vi "Connect References to Bundle By Name.vi"(7 "Sources":refnum<vi>[](array[refnum]), 8 "error in":errorcluster, 9 "BBN Node":refnum<vi>, 10 "SubVI Output Terminal":refnum<vi>) -> (0 "error out":errorcluster, 2 "New Wires":refnum<vi>[](array[refnum]))   [LabVIEW 2015, in "Build Cluster of References__RCF.lvlib"]
doc: "Connects several references to the inputs of a Bundle By Name primitive and aligns them."
uses:
  Build Cluster of References__RCF.lvlib
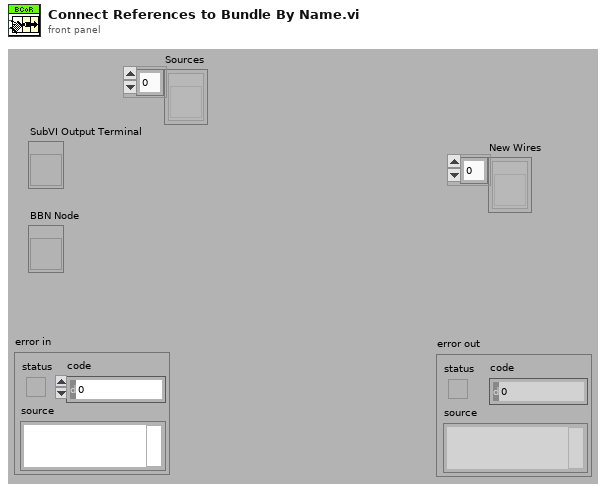
[diagram p1: front panel]
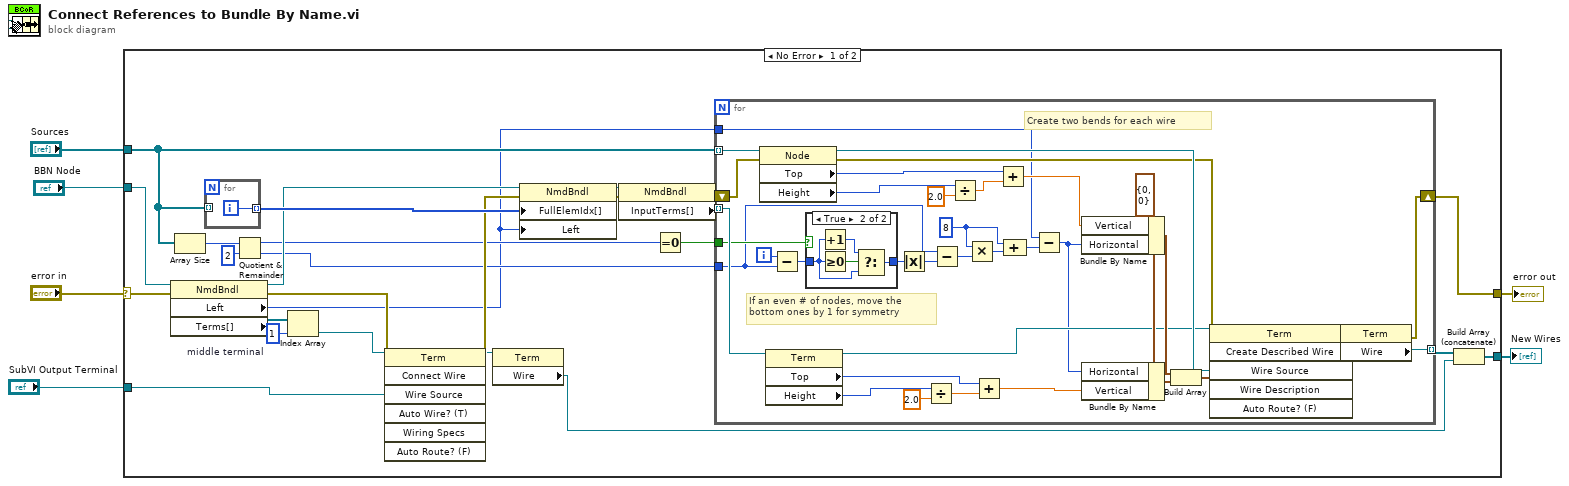
[diagram p0: block diagram]
diagram:
  n1 = case shown="No Error" "error in" {
    selector: "error in" -> [w17 w75]
    tunnel: "Sources" -> [w21 _]
    tunnel: "BBN Node" -> [w19 _]
    tunnel: [w28 w75] -> w3
    tunnel: [w11 _] -> w2
    tunnel: "SubVI Output Terminal" -> [w20 _]
    frame No Error {
      w23 = 1  # middle terminal
      n2 = property class="NmdBndl"(reference=w19, error in=w17) -> (reference out=w14:refnum<vi>, error out=w16:errorcluster, "Left"=w7:i32, "Terms[]"=w22:refnum<vi>[])
      n3 = Array Size(array=w21) -> (size(s)=w9:i32)
      n4 = for {
        tunnel: [w33] -> w18 mode=indexing
        tunnel: w21 -> [_] mode=indexing
        i -> [w33]
      }
      n5 = Quotient & Remainder(x=w9, y=2) -> (x-y*floor(x/y)=w13:i32, floor(x/y)=w8:i32)
      n6 = Index Array(array=w22, index=w23) -> (element=w24:refnum<vi>)
      n7 = invoke class="Term" method="Connect Wire"(reference=w24, error in=w16, "Wire Source"=w20) -> (reference out=w12:refnum<vi>, error out=w15:errorcluster)  [unwired: 4 in, 5 out]
      n8 = property class="Term"(reference=w12) -> ("Wire"=w10:refnum<vi>)  [unwired: 1 in, 2 out]
      n9 = property class="NmdBndl"(reference=w14, error in=w15, "FullElemIdx[]"=w18, "Left"=w7) -> (reference out=w25:refnum<vi>, error out=w26:errorcluster)
      n10 = property class="NmdBndl"(reference=w25, error in=w26) -> (error out=w29:errorcluster, "InputTerms[]"=w32:refnum<vi>[])  [unwired: 1 out]
      n11 = Equal To 0?(x=w13) -> (x = 0?=w27:bool)
      n12 = for {
        tunnel: w32 -> [w54] mode=indexing
        tunnel: w21 -> [w69] mode=indexing
        tunnel: [w58] -> w30 mode=indexing
        tunnel: w8 -> [w35]
        shift-right: [w46] -> w28
        shift-left: w29 -> [w47]
        tunnel: w27 -> [w41]
        tunnel: w7 -> [w39]
        i -> [w38]
        w56 = cluster{"Vertical":i16, "Horizontal":i16} {"Vertical"=0, "Horizontal"=0}
        w43 = 8 ("x")
        # "If an even # of nodes, move the bottom ones by 1 for symmetry"
        # "Create two bends for each wire"
        n13 = property class="Node"(reference=w69, error in=w47) -> (reference out=w57:refnum<vi>, error out=w42:errorcluster, "Top"=w65:i32, "Height"=w68:u32)
        n14 = property class="Term"(reference=w54) -> (reference out=w48:refnum<vi>, "Top"=w51:i32, "Height"=w50:u32)  [unwired: 1 in, 1 out]
        n15 = Subtract(x=w38, y=w35) -> (x-y=w37:i32)
        n16 = case shown="True" w41 {
          tunnel: [w70 w71] -> w40
          tunnel: w37 -> [w70 w73]
          frame False {
          }
          frame True {
            n17 = Increment(x=w73) -> (x+1=w72:i32)
            n18 = Greater Or Equal To 0?(x=w73) -> (x >= 0?=w74:bool)
            n19 = Select(t=w72, s=w74, f=w73) -> (s? t:f=w71:i32)
          }
        }
        n20 = Absolute Value(x=w40) -> (abs(x)=w55:i32)
        n21 = Divide(x=w50, y=2.0) -> (x/y=w53:dbl)
        n22 = Subtract(x=w35, y=w55) -> (x-y=w36:i32)
        n23 = Divide(x=w68, y=2.0) -> (x/y=w66:dbl)
        n24 = Multiply(x=w43, y=w36) -> (x*y=w44:i32)
        n25 = Add(x=w51, y=w53) -> (x+y=w49:dbl)
        n26 = Add(x=w65, y=w66) -> (x+y=w64:dbl)
        n27 = Compound Arithmetic op=ADD(w43, w44) -> (w45:i32)
        n28 = Subtract(x=w39, y=w45) -> (x-y=w34:i32)
        n29 = Bundle By Name(cluster=w56, "Vertical"=w64, "Horizontal"=w34) -> (w63:cluster{"Vertical":i16, "Horizontal":i16})
        n30 = Bundle By Name(cluster=w56, "Horizontal"=w34, "Vertical"=w49) -> (w62:cluster{"Vertical":i16, "Horizontal":i16})
        n31 = Build Array(w63, w62) -> (w61:cluster{"Vertical":i16, "Horizontal":i16}[])
        n32 = invoke class="Term" method="Create Described Wire"(reference=w48, error in=w42, "Wire Source"=w57, "Wire Description"=w61) -> (reference out=w60:refnum<vi>, error out=w59:errorcluster)  [unwired: 2 in, 4 out]
        n33 = property class="Term"(reference=w60, error in=w59) -> (error out=w46:errorcluster, "Wire"=w58:refnum<vi>)  [unwired: 1 out]
      }
      n34 = Build Array (concatenate)(w30, w10) -> (w11:refnum<vi>[])
    }
    frame Error {
    }
  }
  "New Wires" <- w2
  "error out" <- w3
